vi "DecodeBall.vi"(1 "element":u8[](array[numeric]), 3 "Key":i32=-1, 5 "error in (no error)":errorcluster) -> (15 "element 2":u8[](array[numeric]), 19 "error out":errorcluster)   [LabVIEW 2023, in "Referee.lvclass"]
uses:
  Referee.lvclass
  Referee.lvclass/Referee.ctl
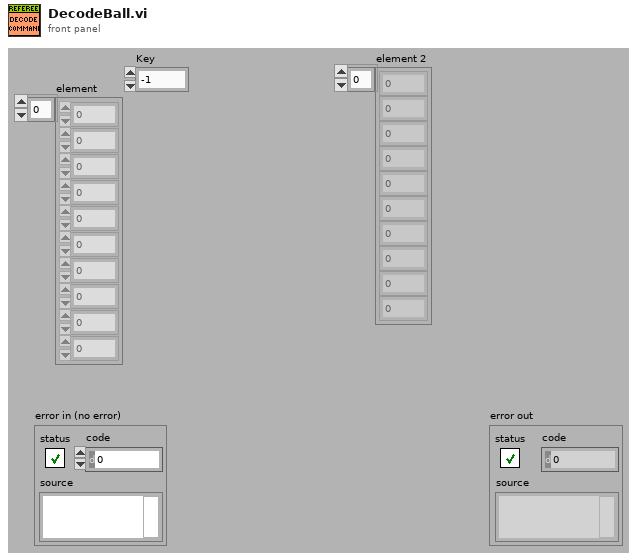
[diagram p1: front panel]
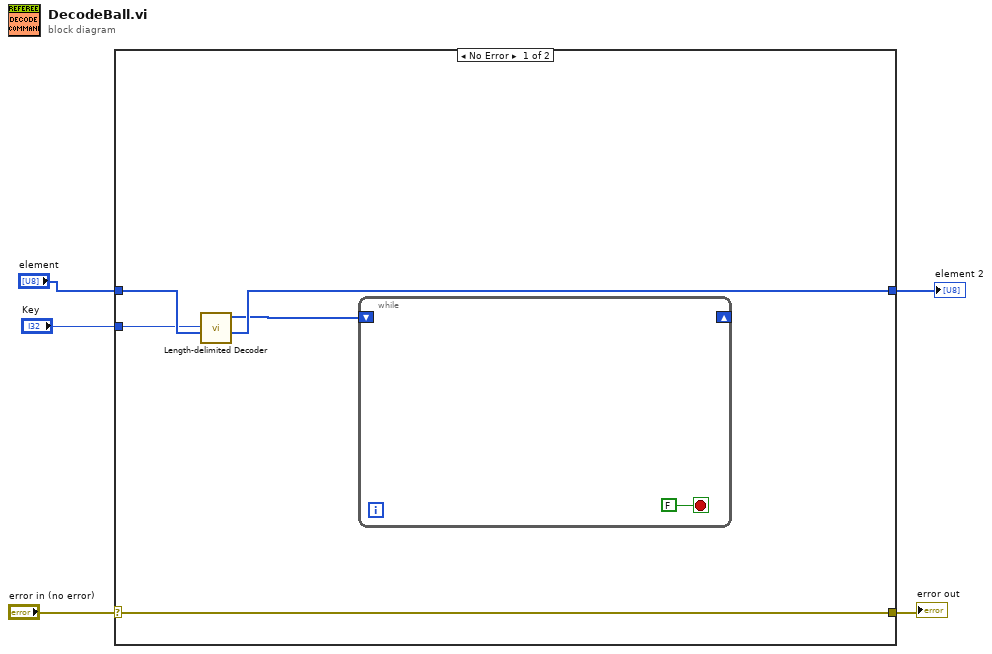
[diagram p0: block diagram]
diagram:
  n1 = case shown="No Error" "error in (no error)" {
    selector: "error in (no error)" -> [w10 w12]
    tunnel: [w10 w12] -> w4
    tunnel: [w8 _] -> w3
    tunnel: "element" -> [w9 _]
    tunnel: "Key" -> [w6 _]
    frame No Error {
      n2 = call "Length-delimited Decoder.vi"("Array"=w9, "Key"=w6) -> ("array w/ subset deleted"=w8:u8[], "Length-delimited"=w7:u8[])  [unwired: 6 in, 2 out]
      n3 = while {
        shift-right: _ -> [_]
        shift-left: w7 -> [_]
        stop <- FALSE stop-if-true
      }
    }
    frame Error {
    }
  }
  "error out" <- w4
  "element 2" <- w3
